vi "NIVETHAN_RAMESH_SERVER.vi"(11 "Television":refnum<k7>(container)) -> ()   [LabVIEW 2021]
panel:
  out "Curtain-Kitchen2":u8(slide) scale=0.0..100.0
  out "Curtain-Kitchen1":u8(slide) scale=0.0..100.0
  out "Curtain-Balcony":u8(slide) scale=0.0..100.0
  out "Curtain-LivingRoom":u8(slide) scale=0.0..100.0
  out "Curtain-Balcony2":u8(slide) scale=0.0..100.0
  out "Curtain-Balcony1":u8(slide) scale=0.0..100.0
  out "Curtain-Bedroom2-2":u8(slide) scale=0.0..100.0
  out "Curtain-Bedroom2-1":u8(slide) scale=0.0..100.0
  out "Curtain-Bedroom1":u8(slide) scale=0.0..100.0
  out "Door-Kitchen2":bool
  out "Door-Balcony":bool
  out "Door-MasterBedroom-Toilet":bool
  out "Door-MasterBedroom":bool
  out "Door-Kitchen-Toilet":bool
  out "Door-Kitchen1":bool
  out "Door-LivingRoom":bool
  out "Door-LivingRoom-Toilet":bool
  out "Door-Bedroom2":bool
  out "Door-Bedroom1":bool
  out "Light-LivingRoom1":bool
  out "Light-Balcony-3":bool
  out "Light-Balcony-2":bool
  out "Light-Kitchen":bool
  out "Light-Balcony-1":bool
  out "Light-Kitchen-Toilet":bool
  out "Light-MasterBedroom2":bool
  out "Light-MasterBedroom1":bool
  out "Light-LivingRoom2":bool
  out "Light-LivingRoom-Toilet":bool
  out "Door-Balcony2":bool
  out "Light-Bedroom1":bool
  out "Light-Bedroom2":bool
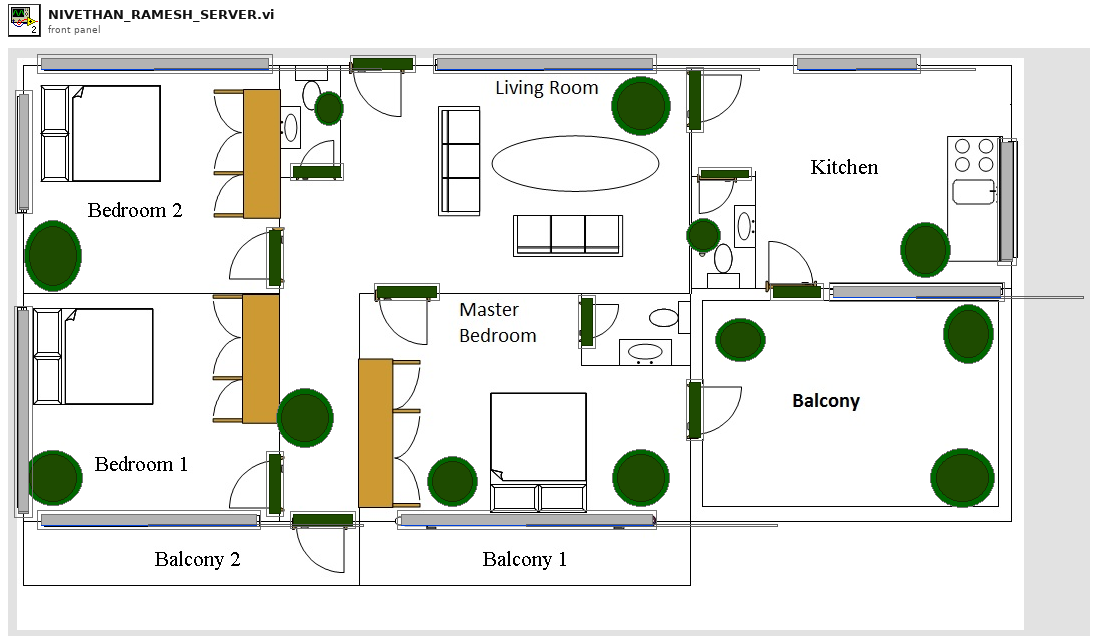
[diagram p1: front panel]
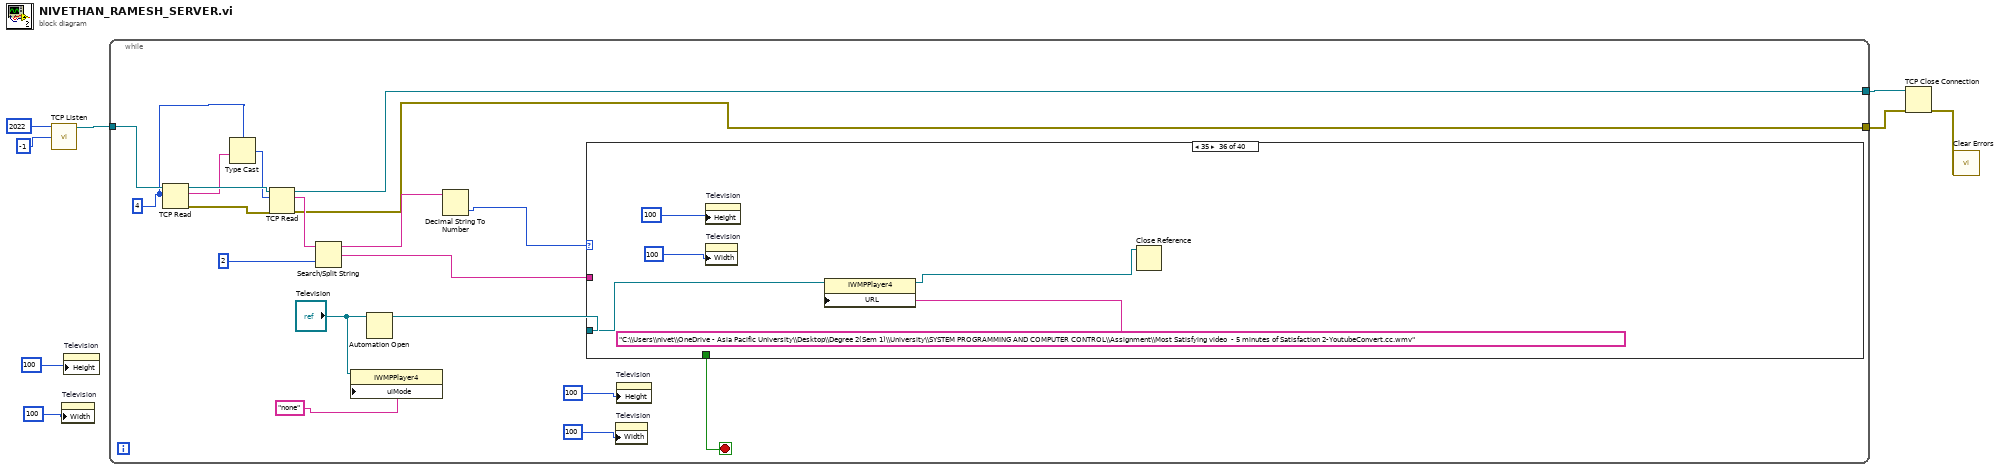
[diagram p0: block diagram]
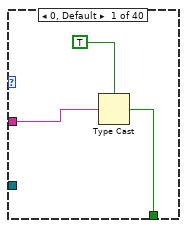
[diagram p2: hidden frame]
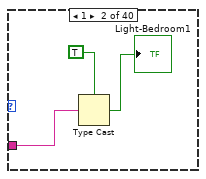
[diagram p3: hidden frame]
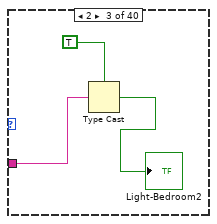
[diagram p4: hidden frame]
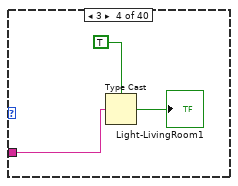
[diagram p5: hidden frame]
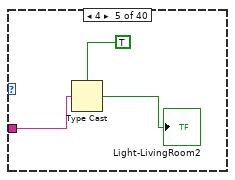
[diagram p6: hidden frame]
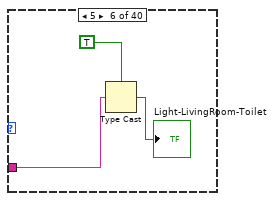
[diagram p7: hidden frame]
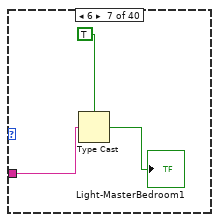
[diagram p8: hidden frame]
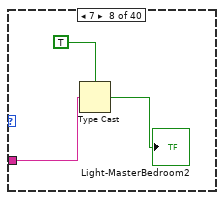
[diagram p9: hidden frame]
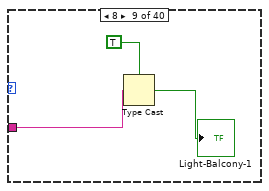
[diagram p10: hidden frame]
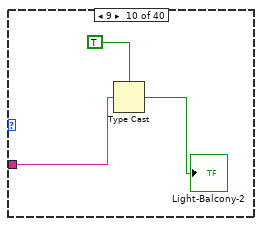
[diagram p11: hidden frame]
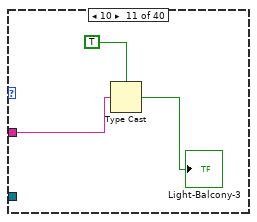
[diagram p12: hidden frame]
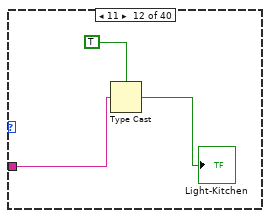
[diagram p13: hidden frame]
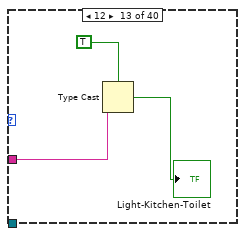
[diagram p14: hidden frame]
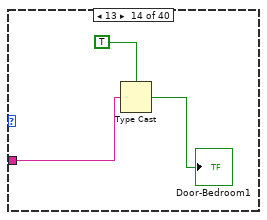
[diagram p15: hidden frame]
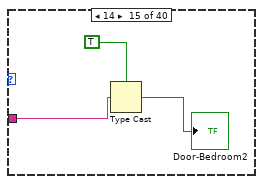
[diagram p16: hidden frame]
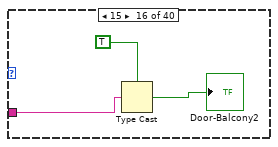
[diagram p17: hidden frame]
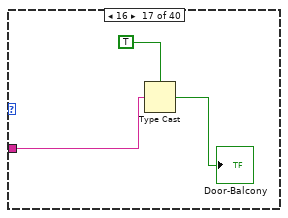
[diagram p18: hidden frame]
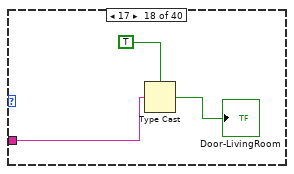
[diagram p19: hidden frame]
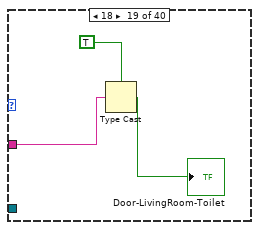
[diagram p20: hidden frame]
diagram:
  n1 = call <vilib>:"TCP Listen.vi"("timeout ms (wait forever: -1)"=-1, "port"=2022) -> ("connection ID"=w6:refnum<k5>)  [unwired: 5 in, 4 out]
  n2 = property on="Television" class="AXCont"("Width"=100) -> ()  [unwired: 2 in, 2 out]
  n3 = property on="Television" class="AXCont"("Height"=100) -> ()  [unwired: 2 in, 2 out]
  n4 = while {
    tunnel: w6 -> [w27]
    tunnel: [w18] -> w5
    tunnel: [w15] -> w4
    stop <- w17 stop-if-true
    w11 = 4
    n5 = TCP Read(connection ID=w27, bytes to read=w11) -> (connection ID out=w26:refnum<k5>, data out=w25:string, error out=w16:errorcluster)  [unwired: 3 in]
    n6 = Type Cast(type=w11, x=w25) -> (*(type *) &x=w24:i32)
    n7 = TCP Read(connection ID=w26, bytes to read=w24, error in (no error)=w16) -> (connection ID out=w18:refnum<k5>, data out=w23:string, error out=w15:errorcluster)  [unwired: 2 in]
    n8 = Search/Split String(string=w23, offset (0)=2) -> (substring before match=w21:string, match + rest of string=w19:string)  [unwired: 1 in, 1 out]
    n9 = property class="IWMPPlayer4"(reference="Television", "uiMode"="none") -> ()  [unwired: 1 in, 2 out]
    n10 = Automation Open(Automation Refnum="Television") -> (Automation Refnum=w14:refnum<k7>)  [unwired: 3 in, 1 out]
    n11 = Decimal String To Number(string=w21) -> (number=w20:i32)  [unwired: 2 in, 1 out]
    n12 = case shown="35" w20 {
      tunnel: w19 -> [w30 w33 w36 w38 w41 w44 w47 w50 w53 w56 w59 w62 w65 w67 w71 w74 w77 w80 w83 w86 w89 w92 w95 w98 w101 w103 w105 w107 w109 w111 w113 w115 w117 _ _ _ _ _ w148 w149]
      tunnel: [w28 _ _ _ _ _ _ _ _ _ _ _ _ _ _ _ _ _ _ _ _ _ _ _ _ _ _ _ _ _ _ _ _ _ _ _ _ _ _ _] -> w17
      tunnel: w14 -> [_ _ _ _ _ _ _ _ _ _ _ _ _ _ _ _ _ _ _ _ _ _ _ _ _ _ _ _ _ _ _ _ _ w121 w127 w132 w137 w142 w147 w150]
      frame 0, Default {
        n13 = Type Cast(type=TRUE, x=w30) -> (*(type *) &x=w28:bool)
      }
      frame 1 {
        n14 = Type Cast(type=TRUE, x=w33) -> (*(type *) &x=→"Light-Bedroom1":bool)
      }
      frame 2 {
        n15 = Type Cast(type=TRUE, x=w36) -> (*(type *) &x=→"Light-Bedroom2":bool)
      }
      frame 3 {
        n16 = Type Cast(type=TRUE, x=w38) -> (*(type *) &x=→"Light-LivingRoom1":bool)
      }
      frame 4 {
        n17 = Type Cast(type=TRUE, x=w41) -> (*(type *) &x=→"Light-LivingRoom2":bool)
      }
      frame 5 {
        n18 = Type Cast(type=TRUE, x=w44) -> (*(type *) &x=→"Light-LivingRoom-Toilet":bool)
      }
      frame 6 {
        n19 = Type Cast(type=TRUE, x=w47) -> (*(type *) &x=→"Light-MasterBedroom1":bool)
      }
      frame 7 {
        n20 = Type Cast(type=TRUE, x=w50) -> (*(type *) &x=→"Light-MasterBedroom2":bool)
      }
      frame 8 {
        n21 = Type Cast(type=TRUE, x=w53) -> (*(type *) &x=→"Light-Balcony-1":bool)
      }
      frame 9 {
        n22 = Type Cast(type=TRUE, x=w56) -> (*(type *) &x=→"Light-Balcony-2":bool)
      }
      frame 10 {
        n23 = Type Cast(type=TRUE, x=w59) -> (*(type *) &x=→"Light-Balcony-3":bool)
      }
      frame 11 {
        n24 = Type Cast(type=TRUE, x=w62) -> (*(type *) &x=→"Light-Kitchen":bool)
      }
      frame 12 {
        n25 = Type Cast(type=TRUE, x=w65) -> (*(type *) &x=→"Light-Kitchen-Toilet":bool)
      }
      frame 13 {
        n26 = Type Cast(type=TRUE, x=w67) -> (*(type *) &x=→"Door-Bedroom1":bool)
      }
      frame 14 {
        n27 = Type Cast(type=TRUE, x=w71) -> (*(type *) &x=→"Door-Bedroom2":bool)
      }
      frame 15 {
        n28 = Type Cast(type=TRUE, x=w74) -> (*(type *) &x=→"Door-Balcony2":bool)
      }
      frame 16 {
        n29 = Type Cast(type=TRUE, x=w77) -> (*(type *) &x=→"Door-Balcony":bool)
      }
      frame 17 {
        n30 = Type Cast(type=TRUE, x=w80) -> (*(type *) &x=→"Door-LivingRoom":bool)
      }
      frame 18 {
        n31 = Type Cast(type=TRUE, x=w83) -> (*(type *) &x=→"Door-LivingRoom-Toilet":bool)
      }
      frame 19 {
        n32 = Type Cast(type=TRUE, x=w86) -> (*(type *) &x=→"Door-MasterBedroom":bool)
      }
      frame 20 {
        n33 = Type Cast(type=TRUE, x=w89) -> (*(type *) &x=→"Door-MasterBedroom-Toilet":bool)
      }
      frame 21 {
        n34 = Type Cast(type=TRUE, x=w92) -> (*(type *) &x=→"Door-Kitchen1":bool)
      }
      frame 22 {
        n35 = Type Cast(type=TRUE, x=w95) -> (*(type *) &x=→"Door-Kitchen2":bool)
      }
      frame 23 {
        n36 = Type Cast(type=TRUE, x=w98) -> (*(type *) &x=→"Door-Kitchen-Toilet":bool)
      }
      frame 24 {
        n37 = Decimal String To Number(string=w101) -> (number=→"Curtain-Bedroom1":i32)  [unwired: 2 in, 1 out]
      }
      frame 25 {
        n38 = Decimal String To Number(string=w103) -> (number=→"Curtain-Bedroom2-1":i32)  [unwired: 2 in, 1 out]
      }
      frame 26 {
        n39 = Decimal String To Number(string=w105) -> (number=→"Curtain-Bedroom2-2":i32)  [unwired: 2 in, 1 out]
      }
      frame 27 {
        n40 = Decimal String To Number(string=w107) -> (number=→"Curtain-Balcony1":i32)  [unwired: 2 in, 1 out]
      }
      frame 28 {
        n41 = Decimal String To Number(string=w109) -> (number=→"Curtain-Balcony2":i32)  [unwired: 2 in, 1 out]
      }
      frame 29 {
        n42 = Decimal String To Number(string=w111) -> (number=→"Curtain-LivingRoom":i32)  [unwired: 2 in, 1 out]
      }
      frame 30 {
        n43 = Decimal String To Number(string=w113) -> (number=→"Curtain-Balcony":i32)  [unwired: 2 in, 1 out]
      }
      frame 31 {
        n44 = Decimal String To Number(string=w115) -> (number=→"Curtain-Kitchen1":i32)  [unwired: 2 in, 1 out]
      }
      frame 32 {
        n45 = Decimal String To Number(string=w117) -> (number=→"Curtain-Kitchen2":i32)  [unwired: 2 in, 1 out]
      }
      frame 33 {
        n46 = property class="IWMPPlayer4"(reference=w121) -> ("controls"=w122:refnum<k7>)  [unwired: 1 in, 2 out]
        n47 = property on="Television" class="AXCont"("Height"=100) -> ()  [unwired: 2 in, 2 out]
        n48 = property on="Television" class="AXCont"("Width"=100) -> ()  [unwired: 2 in, 2 out]
        n49 = invoke class="IWMPControls" method="play"(reference=w122) -> (reference out=w120:refnum<k7>)  [unwired: 2 in, 2 out]
        n50 = Close Reference(reference=w120) -> ()  [unwired: 1 in, 1 out]
      }
      frame 34 {
        n51 = property class="IWMPPlayer4"(reference=w127) -> ("controls"=w124:refnum<k7>)  [unwired: 1 in, 2 out]
        n52 = property on="Television" class="AXCont"("Height"=100) -> ()  [unwired: 2 in, 2 out]
        n53 = property on="Television" class="AXCont"("Width"=100) -> ()  [unwired: 2 in, 2 out]
        n54 = invoke class="IWMPControls" method="stop"(reference=w124) -> (reference out=w123:refnum<k7>)  [unwired: 2 in, 2 out]
        n55 = Close Reference(reference=w123) -> ()  [unwired: 1 in, 1 out]
      }
      frame 35 {
        n56 = property on="Television" class="AXCont"("Height"=100) -> ()  [unwired: 2 in, 2 out]
        n57 = property on="Television" class="AXCont"("Width"=100) -> ()  [unwired: 2 in, 2 out]
        n58 = property class="IWMPPlayer4"(reference=w132, "URL"="C:\\Users\\nivet\\OneDrive - Asia Pacific University\\Desktop\\Degree 2(Sem 1)\\University\\SYSTEM PROGRAMMING AND COMPUTER CONTROL\\Assignment\\Most Satisfying video  - 5 minutes of Satisfaction 2-YoutubeConvert.cc.wmv") -> (reference out=w131:refnum<k7>)  [unwired: 1 in, 1 out]
        n59 = Close Reference(reference=w131) -> ()  [unwired: 1 in, 1 out]
      }
      frame 36 {
        n60 = property on="Television" class="AXCont"("Height"=100) -> ()  [unwired: 2 in, 2 out]
        n61 = property on="Television" class="AXCont"("Width"=100) -> ()  [unwired: 2 in, 2 out]
        n62 = property class="IWMPPlayer4"(reference=w137, "URL"="C:\\Users\\nivet\\OneDrive - Asia Pacific University\\Desktop\\Degree 2(Sem 1)\\University\\SYSTEM PROGRAMMING AND COMPUTER CONTROL\\Assignment\\No Copyright Background Nature Video (No Sound, No Music) - Free Stock Footage-YoutubeConvert.cc.wmv") -> (reference out=w136:refnum<k7>)  [unwired: 1 in, 1 out]
        n63 = Close Reference(reference=w136) -> ()  [unwired: 1 in, 1 out]
      }
      frame 37 {
        n64 = property class="IWMPPlayer4"(reference=w142, "URL"="C:\\Users\\nivet\\OneDrive - Asia Pacific University\\Desktop\\Degree 2(Sem 1)\\University\\SYSTEM PROGRAMMING AND COMPUTER CONTROL\\Assignment\\rose flower time lapse shot slow motion shooted with sony a7s-YoutubeConvert.cc.wmv") -> (reference out=w140:refnum<k7>)  [unwired: 1 in, 1 out]
        n65 = property on="Television" class="AXCont"("Width"=100) -> ()  [unwired: 2 in, 2 out]
        n66 = property on="Television" class="AXCont"("Height"=100) -> ()  [unwired: 2 in, 2 out]
        n67 = Close Reference(reference=w140) -> ()  [unwired: 1 in, 1 out]
      }
      frame 38 {
        n68 = Type Cast(type=TRUE, x=w148) -> (*(type *) &x=w143:bool)
        n69 = property class="IWMPPlayer4"(reference=w147) -> ("settings"=w145:refnum<k7>)  [unwired: 1 in, 2 out]
        n70 = property class="IWMPSettings"(reference=w145, "mute"=w143) -> (reference out=w144:refnum<k7>)  [unwired: 1 in, 1 out]
        n71 = Close Reference(reference=w144) -> ()  [unwired: 1 in, 1 out]
      }
      frame 39 {
        # "Volume control"
        n72 = property class="IWMPPlayer4"(reference=w150) -> ("settings"=w153:refnum<k7>)  [unwired: 1 in, 2 out]
        n73 = Decimal String To Number(string=w149) -> (number=w152:i32)  [unwired: 2 in, 1 out]
        n74 = property class="IWMPSettings"(reference=w153, "volume"=w152) -> (reference out=w151:refnum<k7>)  [unwired: 1 in, 1 out]
        n75 = Close Reference(reference=w151) -> ()  [unwired: 1 in, 1 out]
      }
    }
    n76 = property on="Television" class="AXCont"("Width"=100) -> ()  [unwired: 2 in, 2 out]
    n77 = property on="Television" class="AXCont"("Height"=100) -> ()  [unwired: 2 in, 2 out]
  }
  n78 = TCP Close Connection(connection ID=w5, error in (no error)=w4) -> (error out=w3:errorcluster)  [unwired: 1 in, 1 out]
  n79 = call <vilib>:"Clear Errors.vi"("error in (no error)"=w3) -> ()  [unwired: 5 in, 2 out]
